vi "2014 Ball Detection.vi"() -> ()   [LabVIEW 2015]
uses:
  <vilib>/Rock Robotics/WPI/Camera/WPI_CameraSettings Read MJPG.ctl
  <vilib>/Rock Robotics/WPI/Camera/WPI_CameraImageSize.ctl
panel:
  in  "Std Devs":cluster{"Hue":dbl, "Sat":dbl, "Val":dbl}={"Hue"=4.0, "Sat"=6.0, "Val"=4.0}
  in  "Targets":i32=3
  in  "Area Size Limit %":dbl=0.4 format="%#_13g"
  in  "Instructions:":string="Use the tab immediately below to choose the image source. Update the camera settings or the image directory so that you have images or video to test with.\n\nCalibration:\nYou can update Color Component ranges directly, or by clicking and drawing a line across the upper third of a ball within the image -- example shown below-right.\n\nUse Debugging tab to view intermediate results. Adjust Std Dev multipliers and line to achieve the desired HSV upper and lower threshold limits.\n\nArea Size LImit is used to ignore objects too small or balls too far away to care about.\n\nTargets identifies how many of the top scores to return.\n\nThe Details tab contains center, radius, and score details of each object."
  out "loop time ms":u32
  in  "Score Cutoff":dbl(slide)=70.58823529411765 scale=0.0..100.0
  in  "Color Components":T1={"Hue"={243.23333311080933, 20.233333110809326}, "Sat"={125.60287475585938, 242.93045043945312}, "Val"={83.88507843017578, 225.38158416748047}} {"Val" scale=0.0..255.0; "Sat" scale=0.0..255.0; "Hue" scale=0.0..255.0 scale format="%#_3g"}
  out "Error":bool
  in  "Image Source":enum32{"Files", "Camera"}(tab)
  in  "List of image files":i32(listbox)
  in  "Image Directory":path=path "2014 Vision Target"
  in  "Camera Settings":T2={"fps"=15, "compression"=5, "Image Size"=enum."320x240"}
  in  "Camera IP":string="10.04.19.11"
  in  "Tabbed Info":enum32{"Debugging", "Details"}(tab)
  in  "Annotations":enum16{"None", "Good", "All"}(ring)=enum."Good"
  out "Initial Mask":T4(plugin-control)
  out "Fitted Mask":T4(plugin-control)
  out "Ranked Objects":T5(array[cluster]) {"Score" format="%#.1g"}
  out "Image":T4(plugin-control)
  # "Ranking Colors:\n1. green\n2. cyan\n3. magenta\n4. orange"
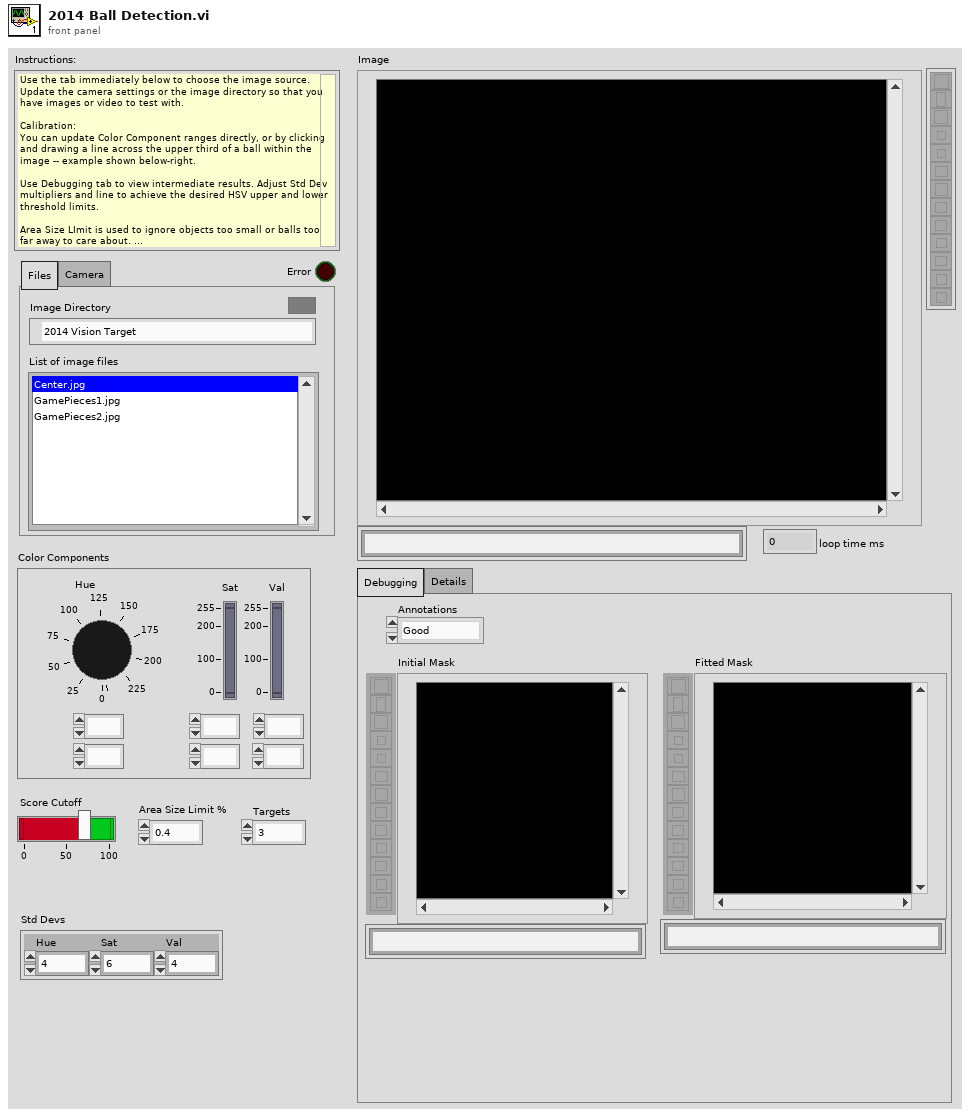
[diagram p1: front panel]
types:
  T1 = cluster{"Hue":cluster{dbl, dbl}, "Sat":cluster{dbl, dbl}, "Val":cluster{dbl, dbl}}
  T2 = typedef "WPI_CameraSettings Read MJPG.ctl" = cluster{"fps":i32, "compression":i32, "Image Size":T3}
  T3 = typedef "WPI_CameraImageSize.ctl" = enum16{"640x480", "320x240", "160x120", "Custom"}
  T4 = typedef "IMAQ Image.ctl" = refnum<image>
  T5 = cluster{"Score":sgl, "Fitted Circle":cluster{"Center":cluster{"X":sgl, "Y":sgl}, "Radius":dbl, "Circle Rect":cluster{"L":sgl, "T":sgl, "R":sgl, "B":sgl}, "Roundness":dbl, "SNR (dB)":dbl}, "Search Rect":cluster{"L":sgl, "T":sgl, "R":sgl, "B":sgl}, "Details":cluster{"Edge":sgl, "Area":sgl, "Circ":sgl, "Diam":sgl}}[]
  T6 = typedef "Image Type" = u32
  T7 = cluster{"Circle Found":bool, "Fitted Circle":cluster{"Center":cluster{"X":sgl, "Y":sgl}, "Radius":dbl, "Center":cluster{"X":sgl, "Y":sgl}, "Radius":dbl, "Roundness":dbl, "Strength":dbl, "SNR (dB)":dbl}, "Array":dbl[], "Sorted Data":dbl[][]}[]
  T8 = cluster{cluster{dbl, dbl}, cluster{dbl, dbl}, cluster{dbl, dbl}}
  T9 = cluster{"Score":dbl, "Fitted Circle":cluster{"Center (Pixels)":cluster{"X":sgl, "Y":sgl}, "Radius (Pixels)":dbl, "Circle Rect":cluster{"Left":sgl, "Top":sgl, "Right":sgl, "Bottom":sgl}, "Roundness (RW)":dbl, "Average SNR (dB)":dbl}, "Search Rect":cluster{"Left":sgl, "Top":sgl, "Right":sgl, "Bottom":sgl}, "Details":cluster{"Edges":sgl, "Circ/Rect":sgl, "Diam/Diam":sgl, "Circularity":sgl}}[]
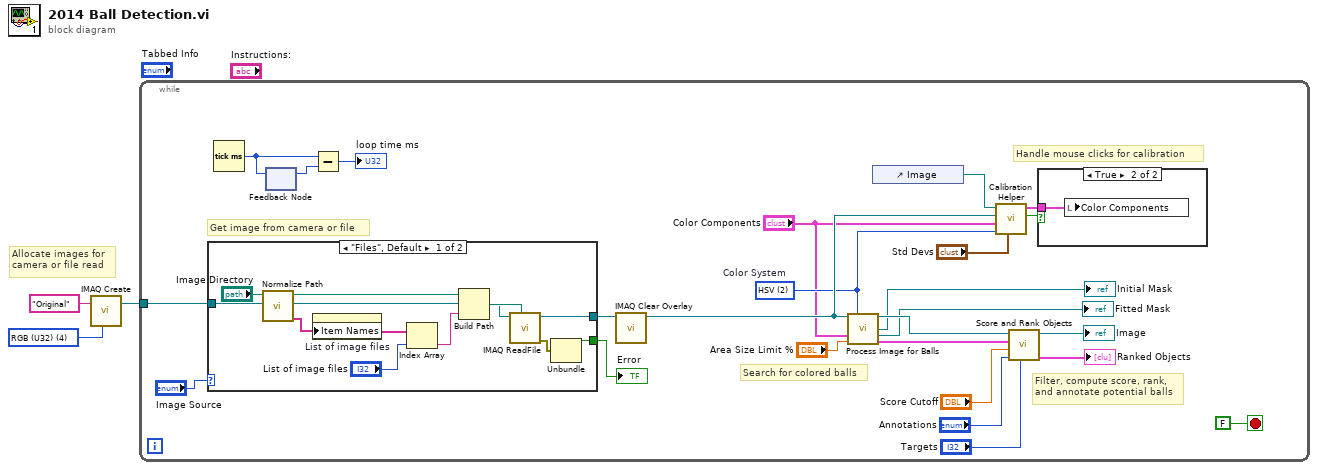
[diagram p0: block diagram]
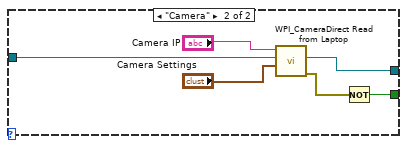
[diagram p3: hidden frame]
diagram:
  w3 = T6 4 items=["Grayscale (U8)", "Grayscale (I16)", "Grayscale (SGL)", "Complex (CSG)", "RGB (U32)", "HSL (U32)", "RGB (U64)", "Grayscale (U16)"] ("Image Type")
  # "Allocate images for\ncamera or file read"
  n1 = call "IMAQ Create"("Image Name"="Original", "Image Type"=w3) -> ("New Image"=w1:T4)  [unwired: 3 in, 1 out]
  n2 = while {
    tunnel: w1 -> [w25]
    stop <- FALSE stop-if-true
    w9 = u16 2 items=["RGB", "HSL", "HSV", "HSI"]  # Color System
    # "Handle mouse clicks for calibration"
    # "Search for colored balls"
    # "Filter, compute score, rank,\nand annotate potential balls"
    # "Get image from camera or file"
    n3 = case shown="\"Files\", Default" "Image Source" {
      tunnel: [w36 w41] -> w28
      tunnel: w25 -> [w35 w43]
      tunnel: [w33 w45] -> w24
      frame "Files", Default {
        n4 = call "Normalize Path.vi"("Image Directory"="Image Directory") -> ("Filenames"=w32:string[], "Path"=w30:path)  [unwired: 9 in]
        n5 = property on="List of image files" class="LstBox (strict)"("Item Names"=w32) -> ()  [unwired: 2 in, 2 out]
        n6 = Index Array(array=w32, index="List of image files") -> (element=w38:string)
        n7 = Build Path(base path=w30, name or relative path=w38) -> (appended path=w37:path)
        n8 = call "IMAQ ReadFile"("File Path"=w37, "Image"=w35) -> ("error out"=w34:errorcluster, "Image Out"=w36:T4)  [unwired: 5 in, 3 out]
        n9 = Unbundle(w34) -> ("status"=w33:bool)  [unwired: 2 out]
      }
      frame "Camera" {
        n10 = call <vilib>:"WPI_CameraDirect Read from Laptop.vi"("Camera Settings"="Camera Settings", "Image"=w43, "address"="Camera IP") -> ("error out"=w40:errorcluster, "Image Out"=w41:T4)  [unwired: 7 in]
        n11 = Not(x=w40) -> (.not. x?=w45:bool)
      }
    }
    "Error" <- w24
    n12 = Tick Count (ms)() -> (millisecond timer value=w23:u32)
    n13 = feedback #1() -> (w22:u32)  [unwired: 1 in]
    n14 = feedback-in #1(w23) -> ()
    n15 = Subtract(x=w23, y=w22) -> (x-y=→"loop time ms":u32)
    n16 = call "IMAQ Clear Overlay"("Image"=w28) -> ("Image Out"=w16:T4)  [unwired: 9 in, 1 out]
    n17 = call "Process Image for Balls.vi"("Src Image"=w16, "Color Mode 2"=w9, "Color"="Color Components", "Area Cutoff %"="Area Size Limit %") -> ("Src Image Out"=w14:T4, "First Threshold"=→"Initial Mask":T4, "Fitted"=→"Fitted Mask":T4, "Potential"=w13:T7)  [unwired: 8 in]
    n18 = control-ref of="Image"() -> (w8:refnum<vi>)
    n19 = call "Calibration Helper.vi"("Std Devs"="Std Devs", "Color Mode"=w9, "Color Components"="Color Components", "Image"=w16, "Image Ctl Refnum"=w8) -> ("Changed"=w5:bool, "output color"=w7:T8)  [unwired: 5 in]
    n20 = call "Score and Rank Objects.vi"("Targets"="Targets", "Annotations"="Annotations", "Score Limit"="Score Cutoff", "Object Info"=w13, "Image in"=w14) -> ("Object Info"=→"Ranked Objects":T9, "Annotated Image"=→"Image":T4)  [unwired: 5 in]
    n21 = case shown="True" w5 {
      tunnel: w7 -> [_ w29]
      frame False {
      }
      frame True {
        n22 = local write "Color Components"(w29) -> ()
      }
    }
  }
